vi "Read OCP Level.vi"(8 "error in":errorcluster, 11 "Electronic Load in":refnum<class "Electronic Load.lvclass">) -> (0 "error out":errorcluster, 2 "OCP Level":dbl, 3 "Electronic Load out":refnum<class "Electronic Load.lvclass">)   [LabVIEW 2019, in "Electronic Load.lvlib" / "Electronic Load.lvclass"]
uses:
  Library/Electronic Load.lvclass
  Library/Electronic Load.lvclass/Electronic Load.ctl
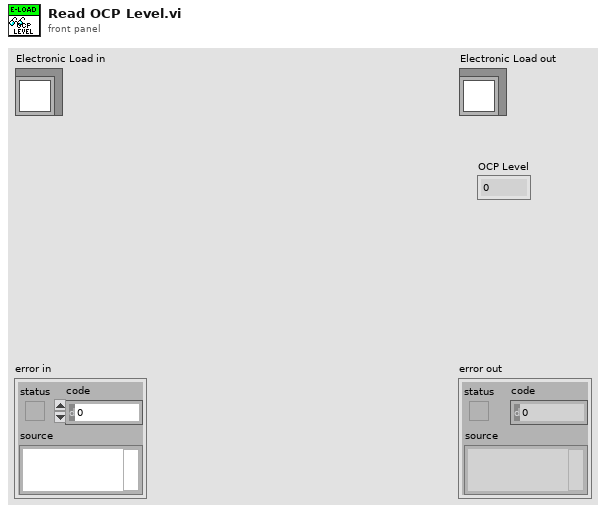
[diagram p1: front panel]
types:
  T1 = typedef "Electronic Load.lvlib/Electronic Load.lvclass/OCP Settings.ctl" = cluster{"OCP_Enabled":bool, "OCP Level":dbl, "OCP Delay":dbl}
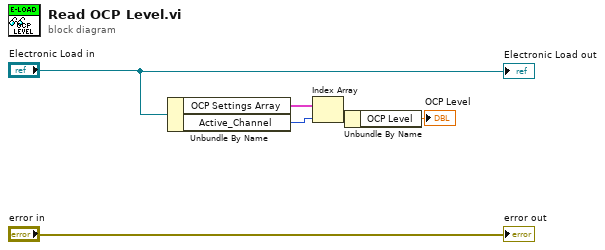
[diagram p0: block diagram]
diagram:
  n1 = Unbundle By Name("Electronic Load in") -> ("OCP Settings Array"=w4:T1[], "Active_Channel"=w3:u32)
  n2 = Index Array(array=w4, index=w3) -> (element=w2:T1)
  n3 = Unbundle By Name(w2) -> ("OCP Level"=→"OCP Level":dbl)
  "error out" <- "error in"
  "Electronic Load out" <- "Electronic Load in"
